vi "QueryNTPparse.vi"(0 "IP Address of NIST Server":string="132.163.4.102", 1 "error in (no error)":errorcluster) -> (2 "NTP Time (20 ns ticks)":u64, 3 "time stamp":timestamp, 4 "error out":errorcluster)   [LabVIEW 2012]
panel:
  out "raw data":string
  # "This is a first draft to query an NTP server (proof of concept).\nhttp://forums.ni.com/ni/board/message?board.id=170&message.id=458949&jump=true"
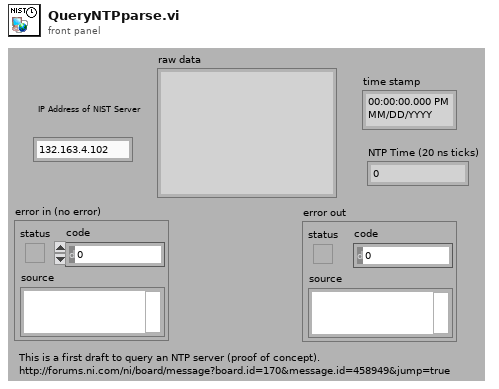
[diagram p1: front panel]
types:
  T1 = cluster{"LI|VM|Mode":u8, "Stratum":u8, "Poll":u8, "Precision":u8, "Root Delay":u32, "Root Dispersion":u32, "Reference Identifier":u32, "Reference Timestamp":fxp<+,64,32>, "Originate Timestamp":fxp<+,64,32>, "Receive Timestamp":fxp<+,64,32>, "Transmit Timestamp":fxp<+,64,32>, "Key Identifier":u32}
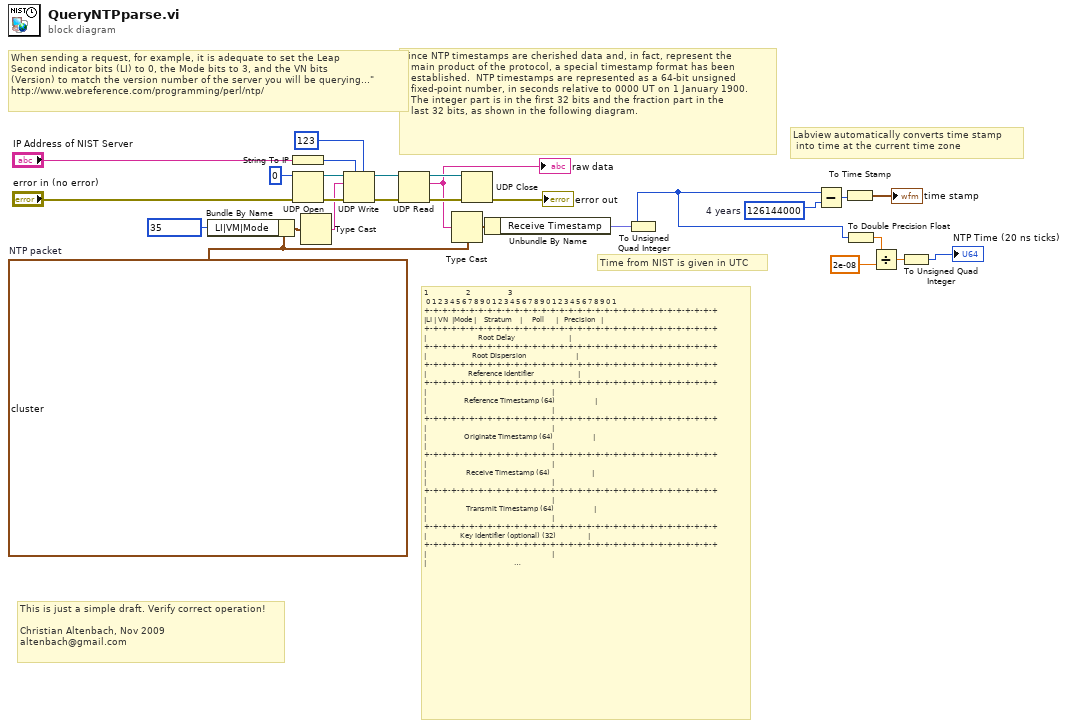
[diagram p0: block diagram]
diagram:
  w7 = u64 126144000  # 4 years
  w10 = T1 {"LI|VM|Mode"=0, "Stratum"=0, "Poll"=0, "Precision"=0, "Root Delay"=0, "Root Dispersion"=0, "Reference Identifier"=0, "Reference Timestamp"=0.0, "Originate Timestamp"=0.0, "Receive Timestamp"=0.0, "Transmit Timestamp"=0.0, "Key Identifier"=0}  # NTP packet
  # "Labview automatically converts time stamp\n into time at the current time zone"
  # "Time from NIST is given in UTC"
  # "This is just a simple draft. Verify correct operation!\n\nChristian Altenbach, Nov 2009\naltenbach@gmail.com"
  # "Since NTP timestamps are cherished data and, in fact, represent the\n   main product of the protocol, a special timestamp format has been\n   established.  NTP timestamps are represented as a 64-bit unsigned\n   fixed-point number, in seconds relative to 0000 UT on 1 January 1900.\n   The integer part is in the first 32 bits and the fraction part in the\n   last 32 bits, as shown in the following diagram."
  # "When sending a request, for example, it is adequate to set the Leap\nSecond indicator bits (LI) to 0, the Mode bits to 3, and the VN bits\n(Version) to match the version number of the server you will be querying...\"\nhttp://www.webreference.com/programming/perl/ntp/"
  # "1                   2                   3\n 0 1 2 3 4 5 6 7 8 9 0 1 2 3 4 5 6 7 8 9 0 1 2 3 4 5 6 7 8 9 0 1\n+-+-+-+-+-+-+-+-+-+-+-+-+-+-+-+-+-+-+-+-+-+-+-+-+-+-+-+-+-+-+-+-+\n|LI | VN  |Mode |    Stratum    |     Poll      |   Precision   |\n+-+-+-+-+-+-+-+-+-+-+-+-+-+-+-+-+-+-+-+-+-+-+-+-+-+-+-+-+-+-+-+-+\n|                          Root Delay                           |\n+-+-+-+-+-+-+-+-+-+-+-+-+-+-+-+-+-+-+-+-+-+-+-+-+-+-+-+-+-+-+-+-+\n|                       Root Dispersion                         |\n+-+-+-+-+-+-+-+-+-+-+-+-+-+-+-+-+-+-+-+-+-+-+-+-+-+-+-+-+-+-+-+-+\n|                     Reference Identifier                      |\n+-+-+-+-+-+-+-+-+-+-+-+-+-+-+-+-+-+-+-+-+-+-+-+-+-+-+-+-+-+-+-+-+\n|                                                               |\n|                   Reference Timestamp (64)                    |\n|                                                               |\n+-+-+-+-+-+-+-+-+-+-+-+-+-+-+-+-+-+-+-+-+-+-+-+-+-+-+-+-+-+-+-+-+\n|                                                               |\n|                   Originate Timestamp (64)                    |\n|                                                               |\n+-+-+-+-+-+-+-+-+-+-+-+-+-+-+-+-+-+-+-+-+-+-+-+-+-+-+-+-+-+-+-+-+\n|                                                               |\n|                    Receive Timestamp (64)                     |\n|                                                               |\n+-+-+-+-+-+-+-+-+-+-+-+-+-+-+-+-+-+-+-+-+-+-+-+-+-+-+-+-+-+-+-+-+\n|                                                               |\n|                    Transmit Timestamp (64)                    |\n|                                                               |\n+-+-+-+-+-+-+-+-+-+-+-+-+-+-+-+-+-+-+-+-+-+-+-+-+-+-+-+-+-+-+-+-+\n|                 Key Identifier (optional) (32)                |\n+-+-+-+-+-+-+-+-+-+-+-+-+-+-+-+-+-+-+-+-+-+-+-+-+-+-+-+-+-+-+-+-+\n|                                                               |\n|                                                               |\n|                 Message Digest (optional) (128)               |\n|                                                               |\n|                                                               |\n+-+-+-+-+-+-+-+-+-+-+-+-+-+-+-+-+-+-+-+-+-+-+-+-+-+-+-+-+-+-+-+-+"
  n1 = Bundle By Name(cluster=w10, "LI|VM|Mode"=u8 35) -> (w8:T1)
  n2 = String To IP(1:"IP Address of NIST Server") -> (0:w22:u32)
  n3 = UDP Open(8:"error in (no error)", 11:u16 0 ("port")) -> (port=w24:refnum<k16>, 0:w21:errorcluster)  [unwired: 3 in, 1 out]
  n4 = Type Cast(x=w8) -> (*(type *) &x=w17:string)  [unwired: 1 in]
  n5 = UDP Write(address=w22, port or service name=u16 123, connection ID=w24, data in=w17, 8:w21) -> (error out=w20:errorcluster, 3:w25:refnum<k16>)  [unwired: 1 in]
  n6 = UDP Read(connection ID=w25, 8:w20) -> (data out=w14:string, error out=w27:errorcluster, 3:w26:refnum<k16>)  [unwired: 2 in, 2 out]
  "raw data" <- w14
  n7 = Type Cast(type=w10, x=w14) -> (*(type *) &x=w13:T1)
  n8 = UDP Close(connection ID=w26, 8:w27) -> (error out=→"error out":errorcluster)  [unwired: 1 out]
  n9 = Unbundle By Name(w13) -> ("Receive Timestamp"=w12:fxp<+,64,32>)
  n10 = To Unsigned Quad Integer(1:w12) -> (0:w1:u64)
  n11 = Subtract(x=w1, y=w7) -> (x-y=w6:u64)
  n12 = To Time Stamp(1:w6) -> (0:→"time stamp":timestamp)
  n13 = To Double Precision Float(number=w1) -> (double precision float=w5:dbl)
  n14 = Divide(x=w5, y=2e-08) -> (x/y=w3:dbl)
  n15 = To Unsigned Quad Integer(1:w3) -> (0:→"NTP Time (20 ns ticks)":u64)
